vi "Detector Get Image.vi"(8 "error in (no error)":errorcluster, 11 "PRIME Detector in":refnum<class "PRIME Detector.lvclass">) -> (0 "error out":errorcluster, 1 "FITS Detector Settings":T2, 2 "Images":T3[](array[typedef]) {"Detector #" items=["None", "YJ", "HK"]}, 3 "PRIME Detector out":refnum<class "PRIME Detector.lvclass">, 4 "Message Log":string, 6 "Detector Files":T1)   [LabVIEW 2021, in "PRIME Detector.lvclass"]
uses:
  PRIME Detector.lvclass
  C:/Development/prime/Prime-RIMAS/Detector/Detector Class/Detector Class.lvclass
  Detector Image typedef cluster.ctl
  RIMAS Observation Config.ctl
  Detector cluster Files.ctl
  Detector Class.lvclass
  PRIME Detector.lvclass/PRIME Detector.ctl
  ed270338-c6d5-43e5-a287-b31ed10c4701.vi
  81b43f0d-8b71-4fcf-9938-3437e86aa932.vi
panel:
  out "Table":string[](array[string])
  # "sec"
  # "sec"
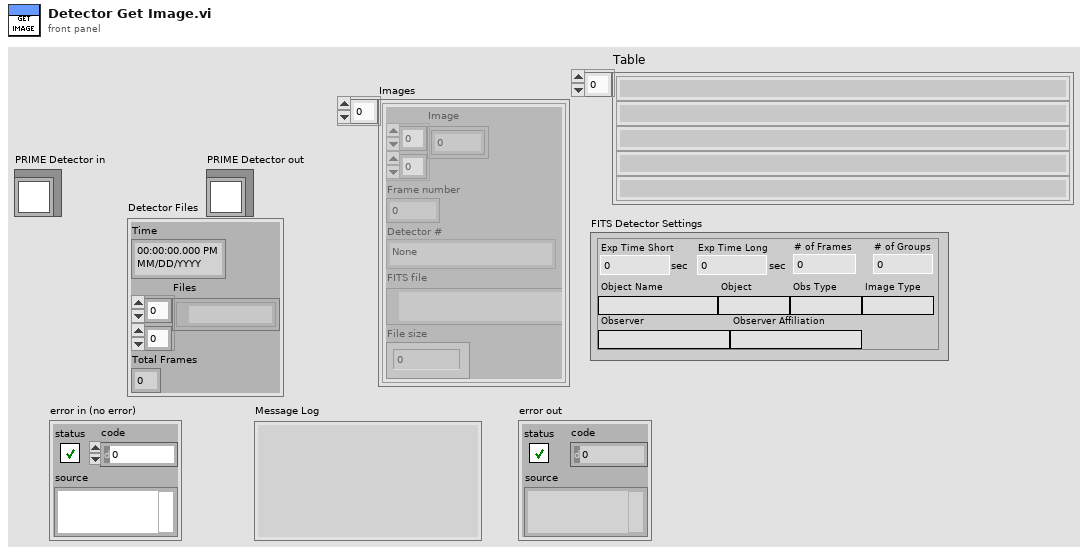
[diagram p1: front panel]
types:
  T1 = typedef "Detector Class.lvclass/Detector cluster Files.ctl" = cluster{"Time":timestamp, "Files":path[][], "Total Frames":i32}
  T2 = typedef "RIMAS Observation Config.ctl" = cluster{"Exp Time Short":dbl, "# of Frames":dbl, "Exp Time Long":dbl, "# of Groups":dbl, "Object Name":string, "Object":string, "Obs Type":string, "Image Type":string, "Observer":string, "Observer Affiliation":string}
  T3 = typedef "Detector Class.lvclass/Detector Image typedef cluster.ctl" = cluster{"Image":sgl[][], "Frame number":i32, "Detector #":u16, "FITS file":path, "File size":i64}
  T4 = typedef "RIMAS Detector Config.ctl" = cluster{"Detector":u16, "Offsets":u16[][], "Detector Computer":T5, "FITS hdr template0":path, "FITS hdr template1":path, "FITS Data File Path":path, "FITS Detector Settings":T2, "Sim Folder":path, "Integration Mode":T6, "Integration Time":dbl, "Frame Int Time":dbl}
  T5 = typedef "RIMAS Detector Server Config.ctl" = cluster{"Machine":string, "Password":string, "FITS File Path":string, "Port":u16, "Header Path":string, "Name":string}
  T6 = typedef "Detector enum Detector Integration Mode.ctl" = enum16{"SSR", "CDS", "MEAN", "MEDIAN", "MODE", "MIIN", "MAX"}
  T7 = typedef "PRIME Detector cluster Status.ctl" = cluster{"Cmd Start Time":timestamp, "Command":string, "Complete?":bool, "Cmd Complete Time":timestamp, "Exp Time Remaining":dbl, "Total Frames":i32, "Exp Frames":cluster{"CAMERA0":string[], "CAMERA1":string[], "CAMERA2":string[], "CAMERA3":string[]}, "Intermediate Frames":cluster{"CAMERA0":string[], "CAMERA1":string[], "CAMERA2":string[], "CAMERA3":string[]}, "Final Reduced Frame":cluster{"CAMERA0":string, "CAMERA1":string, "CAMERA2":string, "CAMERA3":string}}
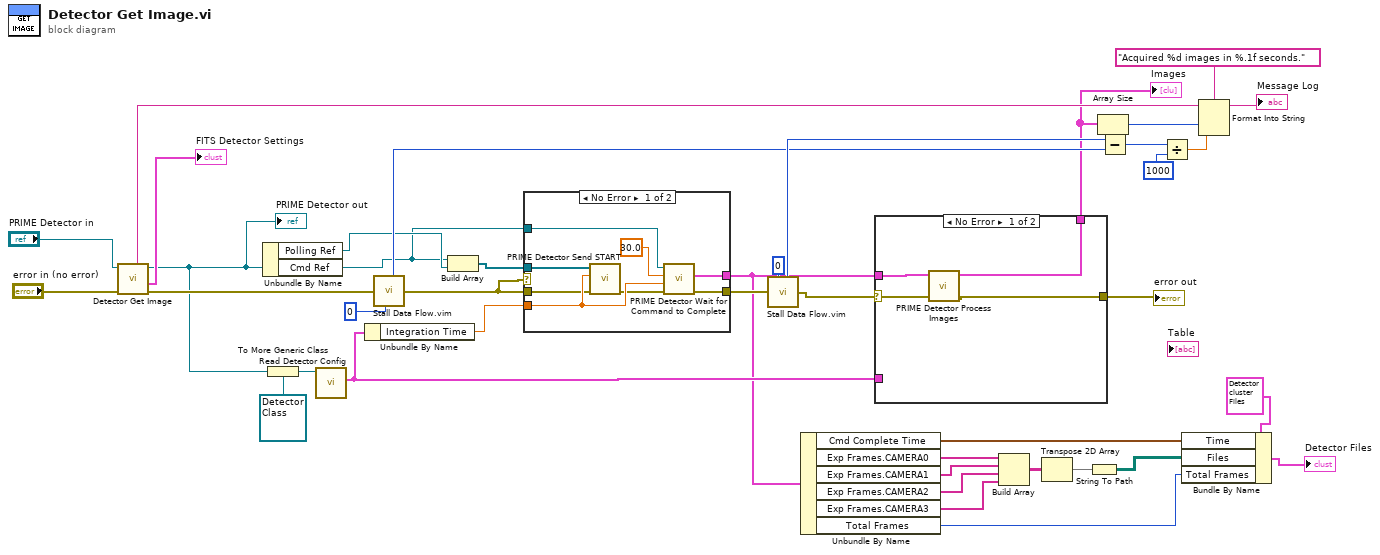
[diagram p0: block diagram]
diagram:
  n1 = call-parent "Detector Get Image.vi"("error in (no error)"="error in (no error)", "Detector Class in"="PRIME Detector in") -> ("error out"=w20:errorcluster, "FITS Detector Settings"=→"FITS Detector Settings":T2, "Detector Class out"=w19:refnum<class "PRIME Detector.lvclass">, "Message Log"=w27:string)  [unwired: 4 in, 2 out]
  "PRIME Detector out" <- w19
  n2 = Unbundle By Name(w19) -> ("Polling Ref"=w22:refnum<k5>, "Cmd Ref"=w14:refnum<k5>)
  n3 = To More Generic Class(target class=refnum<class "Detector Class.lvclass"> refnum ("Detector Class.lvclass"), reference=w19) -> (generic class reference=w37:refnum<class "Detector Class.lvclass">)
  n4 = call-dynamic "Read Detector Config.vi"("Detector Class in"=w37) -> ("Detector Config"=w25:T4)  [unwired: 8 in, 2 out]
  n5 = Unbundle By Name(w25) -> ("Integration Time"=w23:dbl)
  n6 = call "Stall Data Flow.vim"("value in"=w20, "milliseconds to wait"=u32 0) -> ("millisecond timer value"=w34:u32, "value out"=w13:errorcluster)
  n7 = Build Array(w14, w22) -> (w21:refnum<k5>[])
  n8 = case shown="No Error" w13 {
    tunnel: w23 -> [w48 _]
    tunnel: [w45 _] -> w7
    tunnel: w13 -> [w44 w49]
    tunnel: w21 -> [w43 _]
    tunnel: [w42 w49] -> w17
    tunnel: w14 -> [w41 _]
    frame No Error {
      n9 = call "PRIME Detector Send START.vi"("error in (no error)"=w44, "Exposure Time"=w48, "connection ID"=w43) -> ("error out"=w47:errorcluster)  [unwired: 7 in, 1 out]
      n10 = call "PRIME Detector Wait for Command to Complete.vi"("error in (no error)"=w47, "Exp Time"=w48, "timeout (120s)"=30.0, "connection ID"=w41) -> ("error out"=w42:errorcluster, "Status"=w45:T7)  [unwired: 5 in, 1 out]
    }
    frame Error {
    }
  }
  n11 = call "Stall Data Flow.vim"("value in"=w17, "milliseconds to wait"=u32 0) -> ("millisecond timer value"=w35:u32, "value out"=w15:errorcluster)
  n12 = Unbundle By Name(w7) -> ("Cmd Complete Time"=w5:timestamp, "Exp Frames.CAMERA0"=w12:string[], "Exp Frames.CAMERA1"=w11:string[], "Exp Frames.CAMERA2"=w10:string[], "Exp Frames.CAMERA3"=w9:string[], "Total Frames"=w4:i32)
  n13 = case shown="No Error" w15 {
    selector: w15 -> [w51 w54]
    tunnel: w25 -> [_ _]
    tunnel: [w52 _] -> w24
    tunnel: w7 -> [w53 _]
    tunnel: [w50 w54] -> w16
    frame No Error {
      n14 = call "PRIME Detector Process Images.vi"("error in (no error)"=w51, "prime detector status"=w53) -> ("error out"=w50:errorcluster, "Images"=w52:T3[])  [unwired: 8 in]
    }
    frame Error {
    }
  }
  "error out" <- w16
  "Images" <- w24
  n15 = Build Array(w12, w11, w10, w9) -> (w8:string[][])
  n16 = Transpose 2D Array(2D array=w8) -> (transposed array=w3:string[][])
  n17 = String To Path(string=w3) -> (path=w2:path[][])
  n18 = Array Size(array=w24) -> (size(s)=w32:i32)
  n19 = Subtract(x=w35, y=w34) -> (x-y=w31:u32)
  n20 = Divide(x=w31, y=u32 1000) -> (x/y=w29:dbl)
  n21 = Bundle By Name(cluster=T1 {"Time"=timestamp(0 s since 1904-01-01), "Files"=[], "Total Frames"=0} ("Detector Files"), "Time"=w5, "Files"=w2, "Total Frames"=w4) -> (→"Detector Files":T1)
  n22 = Format Into String(format string="Acquired %d images in %.1f seconds.", initial string=w27, w32, w29) -> (resulting string=→"Message Log":string)  [unwired: 1 in, 1 out]
